vi "Finish.vi"   [LabVIEW 2016]
doc: "This VI is called during exit. It can be used to close I/O refnums, save collected data, etc."
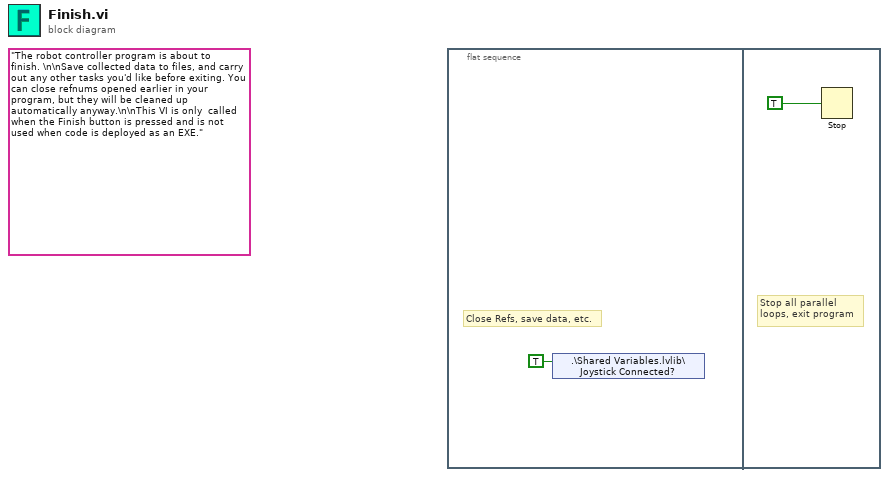
[diagram p0: block diagram]
diagram:
  (unwired) "The robot controller program is about to finish. \n\nSave collected data to files, and carry out any other tasks you'd like before exiting. You can close refnums opened earlier in your program, but they will be cleaned up automatically anyway.\n\nThis VI is only  called when the Finish button is pressed and is not used when code is deployed as an EXE."
  n1 = flat-sequence {
    frame #0 {
      # "Close Refs, save data, etc."
      n2 = shared-variable ".\\Shared Variables.lvlib\\Joystick Connected?"(TRUE ("Joystick Connected?")) -> ()  [unwired: 1 in, 1 out]
    }
    frame #1 {
      # "Stop all parallel\nloops, exit program"
      n3 = Stop(stop? (T)=TRUE ("Quit")) -> ()
    }
  }
